vi "Batch_Create Waveforms_wo_SetID.vi"() -> ()   [LabVIEW 2013]
uses:
  <vilib>/Utility/file.llb/Read From Spreadsheet File (string).vi
panel:
  out "all rows":string[][](array[string])
  in  "Waveform Definition File":path=path "C:/Users/er080167/Documents/XP2100/Documents/Waveforms_to_Create.csv"
  in  "Mode":enum16{"Write", "Read"}(ring)
  in  "Waveform file path":path=path "C:/Users/er080167/Documents/XP2100/Waveforms"
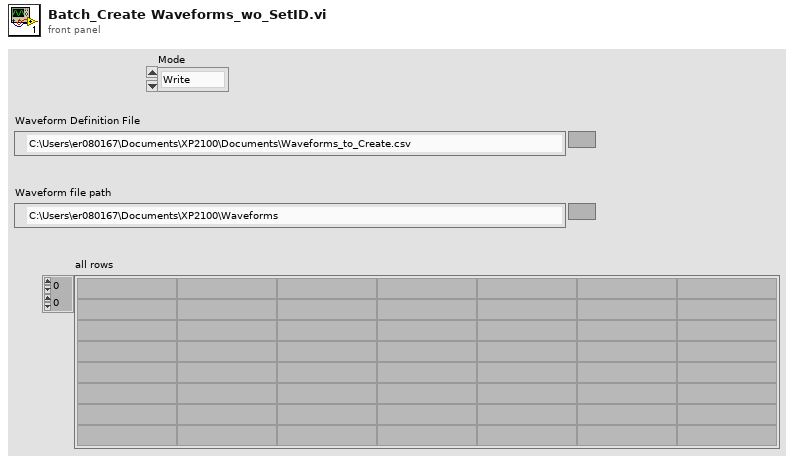
[diagram p1: front panel]
types:
  T1 = cluster{"Slave Address":u8, "Register":u8, "Data":u8}
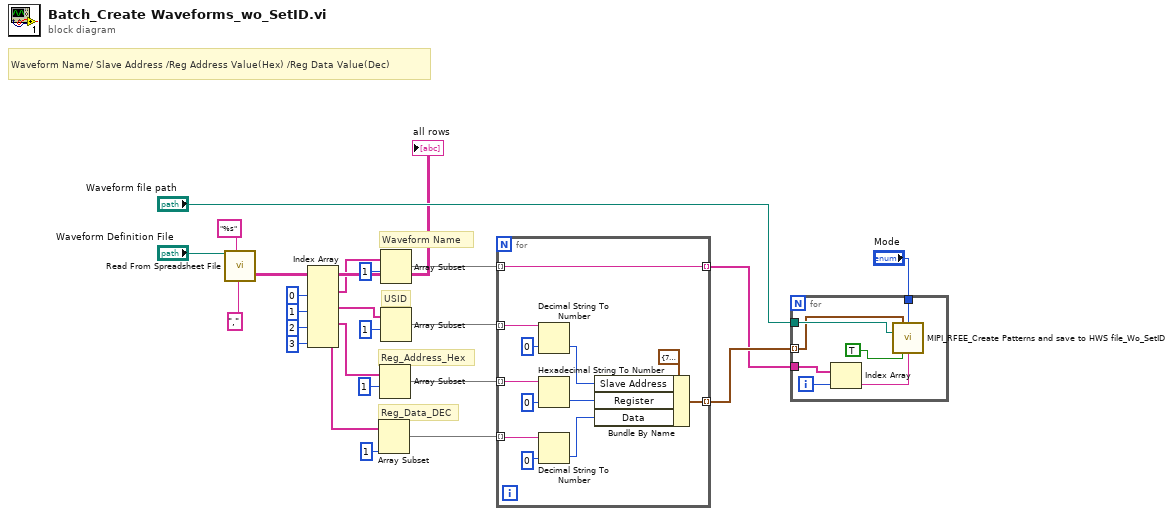
[diagram p0: block diagram]
diagram:
  # "Reg_Data_DEC"
  # "Reg_Address_Hex"
  # "USID"
  # "Waveform Name"
  # "Waveform Name/\tSlave Address\t/Reg Address Value(Hex)\t/Reg Data Value(Dec)"
  n1 = call-poly <vilib>:"Read From Spreadsheet File.vi"("delimiter (\\t)"="," ("delimiter (\\t)"), "format (%s)"="%s", "file path (dialog if empty)"="Waveform Definition File") -> ("all rows"=w22:string[][])  [unwired: 4 in, 4 out]
  "all rows" <- w22
  n2 = Index Array(array=w22, index (col) #1=0 ("disabled index (col)"), index (col) #2=1 ("index (col)"), index (col) #3=2 ("index (col)"), index (col) #4=3 ("index (col)")) -> (element #1=w17:string[], element #2=w13:string[], element #3=w10:string[], element #4=w6:string[])  [unwired: 4 in]
  n3 = Array Subset(array=w6, index=1) -> (w5:string[])  [unwired: 1 in]
  n4 = Array Subset(array=w10, index=1) -> (w9:string[])  [unwired: 1 in]
  n5 = Array Subset(array=w17, index=1) -> (w15:string[])  [unwired: 1 in]
  n6 = Array Subset(array=w13, index=1) -> (w14:string[])  [unwired: 1 in]
  n7 = for {
    tunnel: w15 -> [w28] mode=indexing
    tunnel: w14 -> [w30] mode=indexing
    tunnel: [w31] -> w4 mode=indexing
    tunnel: w9 -> [w29] mode=indexing
    tunnel: [w28] -> w3 mode=indexing
    tunnel: w5 -> [w27] mode=indexing
    n8 = Decimal String To Number(string=w30, default (0L)=u8 0 ("Slave Address")) -> (number=w32:u8)  [unwired: 1 in, 1 out]
    n9 = Hexadecimal String To Number(string=w29, default (0uL)=u8 0 ("Register")) -> (number=w34:u8)  [unwired: 1 in, 1 out]
    n10 = Decimal String To Number(string=w27, default (0L)=u8 0 ("Data")) -> (number=w25:u8)  [unwired: 1 in, 1 out]
    n11 = Bundle By Name(cluster=T1 {"Slave Address"=7, "Register"=65, "Data"=3} ("Register Read/Write"), "Slave Address"=w32, "Register"=w34, "Data"=w25) -> (w31:T1)
  }
  n12 = for {
    tunnel: "Waveform file path" -> [w39]
    tunnel: "Mode" -> [w38]
    tunnel: w4 -> [w37] mode=indexing
    tunnel: w3 -> [w42]
    i -> [w43]
    n13 = Index Array(array=w42, index=w43) -> (element=w40:string)
    n14 = call "MIPI_RFEE_Create Patterns and save to HWS file_Wo_SetID.vi"("Write Data"=w37, "Mode"=w38, "file path"=w39, "Save .HWS?"=TRUE, "Filename"=w40) -> ()  [unwired: 11 in]
  }
